vi "S2C_LoadSubScript.vi"(6 "Insert?":bool, 7 "ItemTag":string, 8 "Error In":errorcluster, 9 "Row":i32, 10 "FuncData":string[](array[string]), 11 "TblData In":string[][](array[string])) -> (0 "Error Out":errorcluster, 3 "TblData Out":string[][](array[string]))   [LabVIEW 2015]
doc: "Adds a new blank row to the script build table if there is currently not one, and sets the Top-left cell to show the new row."
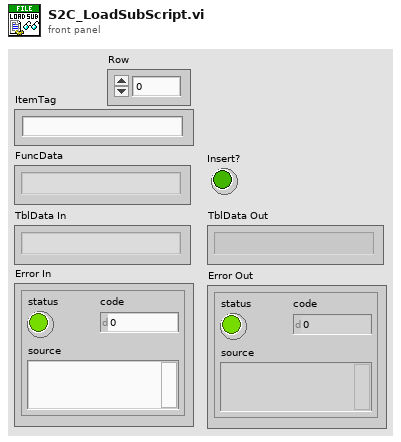
[diagram p1: front panel]
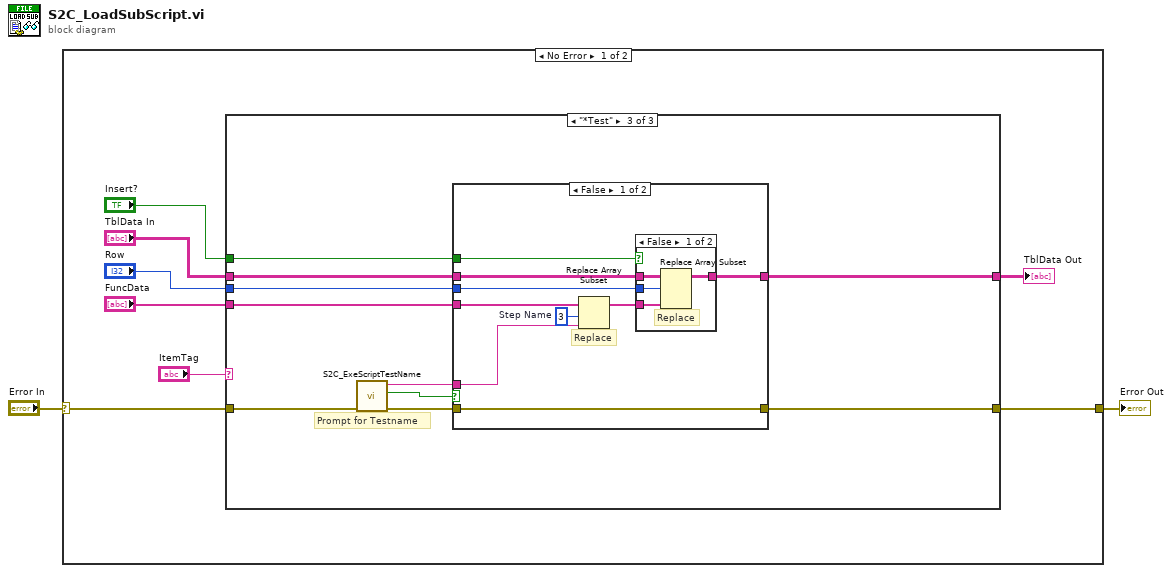
[diagram p0: block diagram]
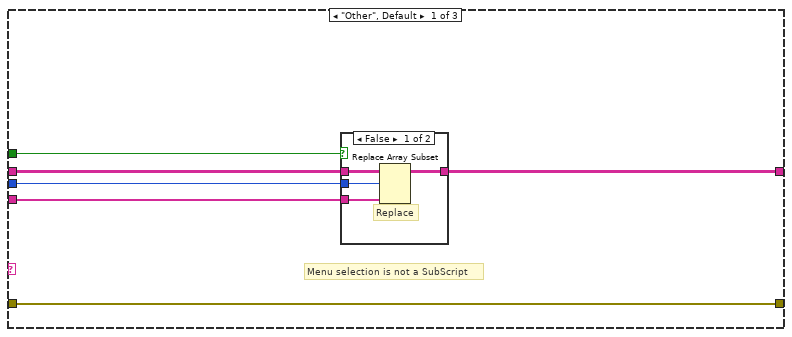
[diagram p2: hidden frame]
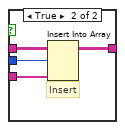
[diagram p3: hidden frame]
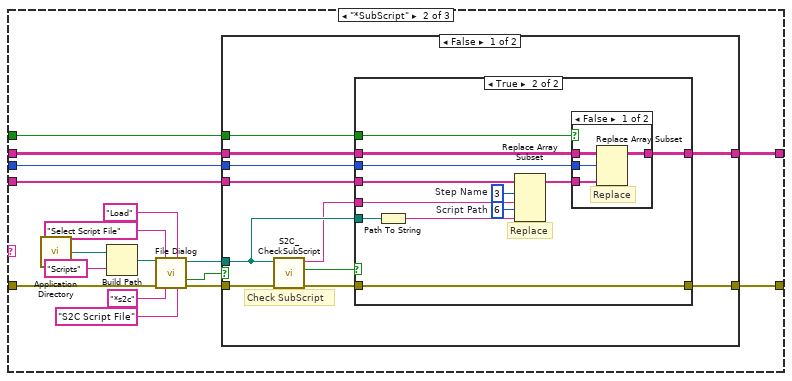
[diagram p4: hidden frame]
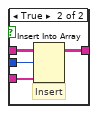
[diagram p6: hidden frame]
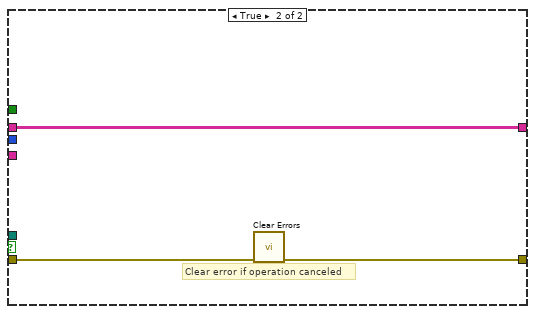
[diagram p7: hidden frame]
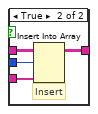
[diagram p8: hidden frame]
diagram:
  n1 = case shown="No Error" "Error In" {
    selector: "Error In" -> [w10 w107]
    tunnel: [w9 w107] -> w1
    frame No Error {
      n2 = case shown="\"*Test\"" "ItemTag" {
        tunnel: w10 -> [w11 w41 w82]
        tunnel: [w11 w32 w78] -> w9
        tunnel: "Insert?" -> [w16 w29 w87]
        tunnel: "TblData In" -> [w15 w28 w86]
        tunnel: "Row" -> [w14 w27 w85]
        tunnel: "FuncData" -> [w13 w26 w84]
        tunnel: [w12 w25 w83] -> w3
        frame "Other", Default {
          # "Menu selection is not a SubScript"
          n3 = case shown="False" w16 {
            tunnel: w15 -> [w20 w24]
            tunnel: w13 -> [w17 w23]
            tunnel: w14 -> [w18 w22]
            tunnel: [w19 w21] -> w12
            frame False {
              # "Replace"
              n4 = Replace Array Subset(array=w20, new element=w17, index (row)=w18) -> (w19:string[][])  [unwired: 1 in]
            }
            frame True {
              # "Insert"
              n5 = Insert Into Array(array=w24, index (row)=w22, new element=w23) -> (w21:string[][])  [unwired: 1 in]
            }
          }
        }
        frame "*SubScript" {
          n6 = call <vilib>:"Application Directory.vi"() -> ("Application Directory"=w39:path)
          n7 = Build Path(base path=w39, name or relative path="Scripts") -> (appended path=w37:path)
          n8 = call "File Dialog"("start path"=w37, "prompt"="Select Script File", "button label"="Load", "error in"=w41, "pattern (all files)"="*s2c", "pattern label"="S2C Script File") -> ("selected path"=w31:path, "cancelled"=w30:bool, "error out"=w33:errorcluster)  [unwired: 6 in, 1 out]
          n9 = case shown="False" w30 {
            tunnel: w33 -> [w46 w77]
            tunnel: w31 -> [w44 _]
            tunnel: [w52 w76] -> w32
            tunnel: w29 -> [w51 _]
            tunnel: w28 -> [w50 w75]
            tunnel: w27 -> [w49 _]
            tunnel: w26 -> [w48 _]
            tunnel: [w47 w75] -> w25
            frame False {
              # "Check SubScript"
              n10 = call "S2C_CheckSubScript.vi"("Error In"=w46, "Path"=w44) -> ("Error Out"=w45:errorcluster, "Continue?"=w42:bool, "Filename"=w43:string)  [unwired: 7 in]
              n11 = case shown="True" w42 {
                tunnel: [w53 w55] -> w52
                tunnel: w45 -> [w53 w55]
                tunnel: w51 -> [_ w66]
                tunnel: w50 -> [w54 w65]
                tunnel: w49 -> [_ w64]
                tunnel: w48 -> [_ w63]
                tunnel: [w54 w62] -> w47
                tunnel: w43 -> [_ w57]
                tunnel: w44 -> [_ w56]
                frame False {
                  # "Issue with SubScript encountered"
                }
                frame True {
                  w60 = 6  # Script Path
                  w61 = 3  # Step Name
                  # "Replace"
                  n12 = Path To String(path=w56) -> (string=w59:string)
                  n13 = Replace Array Subset(array=w63, new element #1=w57, index #1=w61, new element #2=w59, index #2=w60) -> (w58:string[])
                  n14 = case shown="False" w66 {
                    tunnel: w65 -> [w70 w74]
                    tunnel: w58 -> [w67 w73]
                    tunnel: w64 -> [w68 w72]
                    tunnel: [w69 w71] -> w62
                    frame False {
                      # "Replace"
                      n15 = Replace Array Subset(array=w70, new element=w67, index (row)=w68) -> (w69:string[][])  [unwired: 1 in]
                    }
                    frame True {
                      # "Insert"
                      n16 = Insert Into Array(array=w74, index (row)=w72, new element=w73) -> (w71:string[][])  [unwired: 1 in]
                    }
                  }
                }
              }
            }
            frame True {
              # "Clear error if operation canceled"
              n17 = call <vilib>:"Clear Errors.vi"("error in (no error)"=w77) -> ("error out"=w76:errorcluster)  [unwired: 5 in, 1 out]
            }
          }
        }
        frame "*Test" {
          # "Prompt for Testname"
          n18 = call "S2C_ExeScriptTestName.vi"("Error In"=w82) -> ("Error Out"=w80:errorcluster, "Canceled?"=w79:bool, "Name Out"=w81:string)  [unwired: 8 in]
          n19 = case shown="False" w79 {
            tunnel: w87 -> [w96 _]
            tunnel: w86 -> [w95 w106]
            tunnel: w85 -> [w94 _]
            tunnel: w84 -> [w93 _]
            tunnel: [w92 w106] -> w83
            tunnel: w81 -> [w89 _]
            tunnel: w80 -> [w88 w105]
            tunnel: [w88 w105] -> w78
            frame False {
              w91 = 3  # Step Name
              # "Replace"
              n20 = Replace Array Subset(array=w93, new element=w89, index=w91) -> (w90:string[])
              n21 = case shown="False" w96 {
                tunnel: w95 -> [w100 w104]
                tunnel: w90 -> [w97 w103]
                tunnel: w94 -> [w98 w102]
                tunnel: [w99 w101] -> w92
                frame False {
                  # "Replace"
                  n22 = Replace Array Subset(array=w100, new element=w97, index (row)=w98) -> (w99:string[][])  [unwired: 1 in]
                }
                frame True {
                  # "Insert"
                  n23 = Insert Into Array(array=w104, index (row)=w102, new element=w103) -> (w101:string[][])  [unwired: 1 in]
                }
              }
            }
            frame True {
              # "Operation Cancelled"
            }
          }
        }
      }
      "TblData Out" <- w3
    }
    frame Error {
    }
  }
  "Error Out" <- w1
